vi "Write Binary File With Some Samples.vi"() -> ()   [LabVIEW 2014]
panel:
  in  "file path (use dialog)":path=path "C:/Users/Simon Gurfunkel/Documents/LabVIEW_projects/Arduino-projects/LICENSE.txt"
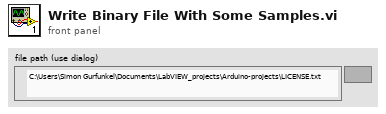
[diagram p1: front panel]
types:
  T1 = enum16{"open", "replace", "create", "open or create", "replace or create", "replace or create with confirmation"}
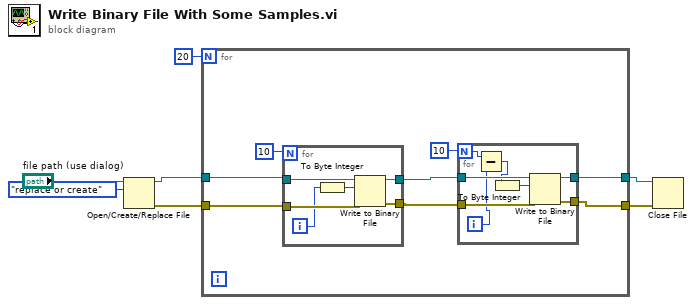
[diagram p0: block diagram]
diagram:
  n1 = Open/Create/Replace File(file path (use dialog)="file path (use dialog)", operation (0:open)=T1."replace or create") -> (refnum out=w4:refnum<file>, error out=w5:errorcluster)  [unwired: 4 in, 1 out]
  n2 = for {
    N: 20 -> [_]
    tunnel: w4 -> [w13]
    tunnel: [w8] -> w2
    tunnel: w5 -> [w15]
    tunnel: [w9] -> w3
    n3 = for {
      N: 10 -> [_]
      tunnel: w15 -> [w29]
      tunnel: [w28] -> w10
      tunnel: w13 -> [w27]
      tunnel: [w24] -> w11
      i -> [w25]
      n4 = To Byte Integer(number=w25) -> (8bit integer=w26:i8)
      n5 = Write to Binary File(file (use dialog)=w27, data=w26, error in=w29) -> (refnum out=w24:refnum<file>, error out=w28:errorcluster)  [unwired: 3 in, 1 out]
    }
    n6 = for {
      N: 10 -> [w18]
      tunnel: w10 -> [w23]
      tunnel: [w22] -> w9
      tunnel: w11 -> [w21]
      tunnel: [w16] -> w8
      i -> [w17]
      n7 = Subtract(x=w18, y=w17) -> (x-y=w19:i32)
      n8 = To Byte Integer(number=w19) -> (8bit integer=w20:i8)
      n9 = Write to Binary File(file (use dialog)=w21, data=w20, error in=w23) -> (refnum out=w16:refnum<file>, error out=w22:errorcluster)  [unwired: 3 in, 1 out]
    }
  }
  n10 = Close File(refnum=w2, error in=w3) -> ()  [unwired: 2 out]
